vi "CAPTH-Simulplot.vi"(10 "ID":i32, 11 "User":string) -> ()   [LabVIEW 2020]
uses:
  SUV/LV Source/SUV VIs/Typedefs/SUV-Experiment State.ctl
panel:
  out "Label":string="2-9   \r2-1   \r2-0   \r"
  out "AUDIOGRAM":cluster{ext[], ext[]}[](graph)
  in  "Run list":string caption="Type run#'s here -  \"xx;yy;zz\""
  in  "Exit":bool
  in  "Go":bool
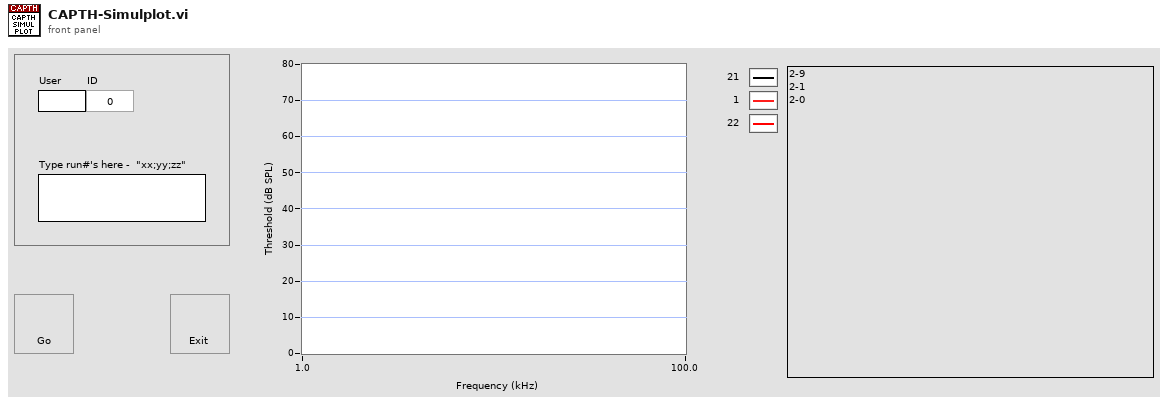
[diagram p1: front panel]
types:
  T1 = typedef "SUV-Experiment State.ctl" = cluster{"User":string, "ID":i32, "Folder":path, "Run":cluster{"DP":i32, "CAP":i32, "SU":i32}, "StateFile":path, "Right":string, "Left":string, "Unit":i32}
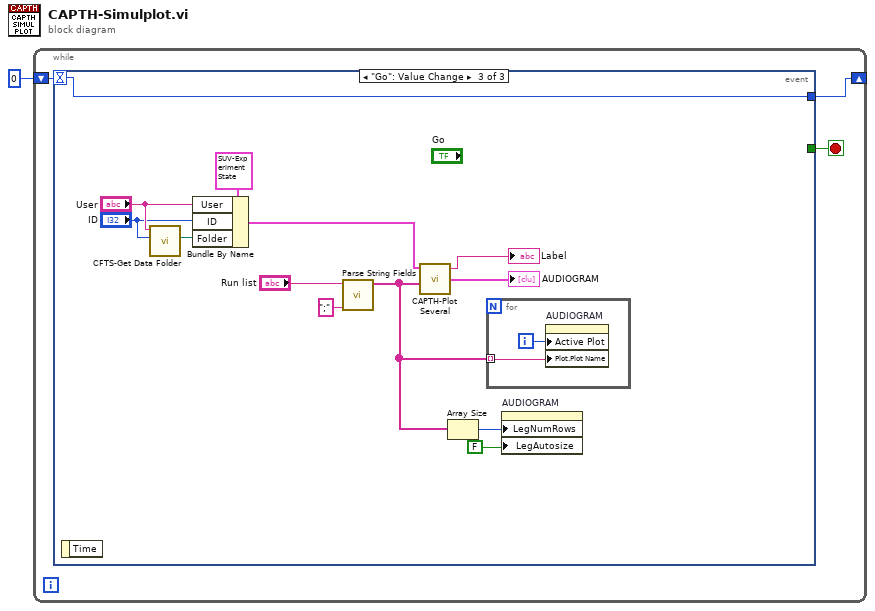
[diagram p0: block diagram]
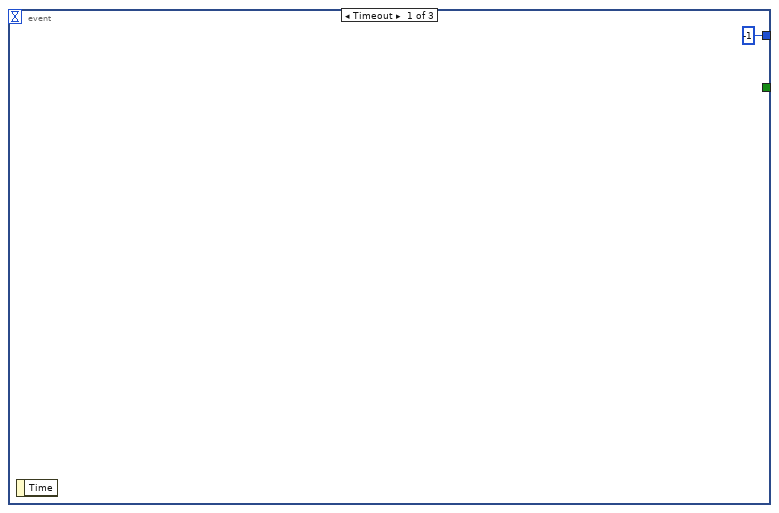
[diagram p2: hidden frame]
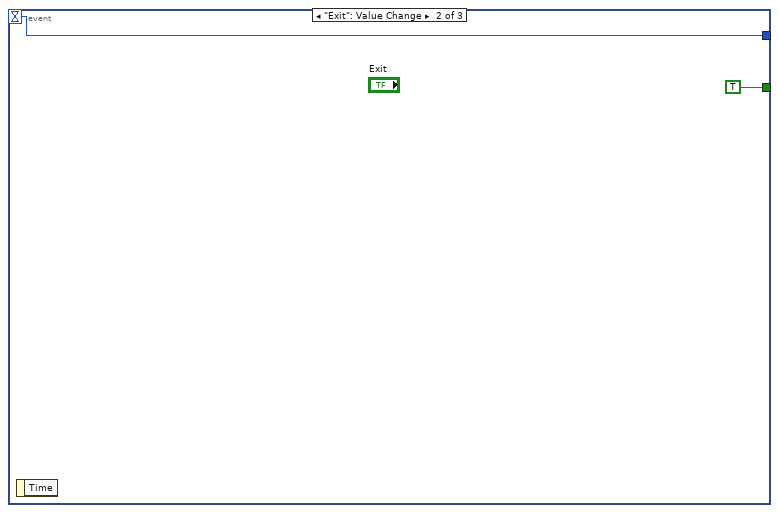
[diagram p3: hidden frame]
diagram:
  n1 = while {
    shift-right: [w3] -> _
    shift-left: 0 -> [w4]
    stop <- w2 stop-if-true
    n2 = event shown="[2] \"Go\": Value Change" {
      selector: _ -> [_ _ _]
      dyn-events: _ -> [_ _ _]
      timeout: w4 -> [_ w7 w15]
      tunnel: [-1 w7 w15] -> w3
      tunnel: [_ TRUE _] -> w2
      event Timeout {
        n3 = event-data() -> ()  [unwired: 1 in, 1 out]
      }
      event "Exit": Value Change {
        n4 = event-data() -> ()  [unwired: 1 in, 1 out]
      }
      event "Go": Value Change {
        n5 = event-data() -> ()  [unwired: 1 in, 1 out]
        n6 = call "CFTS-Get Data Folder.vi"("Number"="ID", "Experimenter"="User") -> ("Data folder"=w17:path)  [unwired: 8 in, 1 out]
        n7 = Bundle By Name(cluster=T1 {"User"="", "ID"=0, "Folder"=path "", "Run"={"DP"=0, "CAP"=0, "SU"=0}, "StateFile"=path "", "Right"="", "Left"="", "Unit"=0} ("State"), "User"="User", "ID"="ID", "Folder"=w17) -> (w16:T1)
        n8 = call "Parse String Fields.vi"("Separator"=";", "String"="Run list") -> ("Fields"=w13:string[])  [unwired: 8 in, 1 out]
        n9 = call "CAPTH-Plot Several.vi"("State"=w16, "Run List"=w13) -> ("Label"=→"Label":string, "FINAL GRAPH"=→"AUDIOGRAM":cluster{ext[], ext[]}[])  [unwired: 4 in]
        n10 = Array Size(array=w13) -> (size(s)=w10:i32)
        n11 = for {
          tunnel: w13 -> [w22] mode=indexing
          i -> [w21]
          n12 = property on="AUDIOGRAM" class="XYGraph (strict)"("Active Plot"=w21, "Plot.Plot Name"=w22) -> ()  [unwired: 2 in, 2 out]
        }
        n13 = property on="AUDIOGRAM" class="XYGraph (strict)"("LegNumRows"=w10, "LegAutosize"=FALSE ("Legend:Autosize")) -> ()  [unwired: 2 in, 2 out]
      }
    }
  }
